vi "Conv AB to enum.vi"(8 "Error In":errorcluster, 11 "Inputs":T2) -> (0 "Error Out":errorcluster, 3 "Input State":T1)   [LabVIEW 2018]
doc: "This VI transforms the input cluster into an enumerated type for specifying the state of the inputs A and B."
uses:
  controls/Cluster for displaying  ABR switch states.ctl
  Enum Defining AB State.ctl
  controls/Enum Defining FSM State.ctl
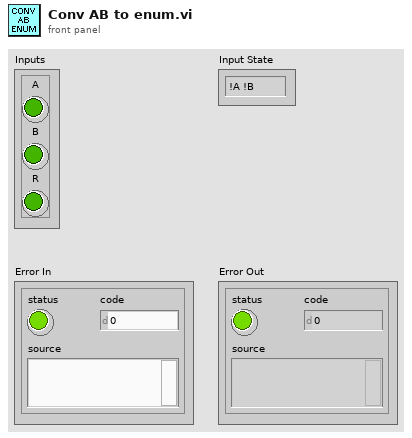
[diagram p1: front panel]
types:
  T1 = typedef "Enum Defining AB State.ctl" = enum16{"!A !B", "!A  B", " A !B", " A B"}
  T2 = typedef "Cluster for displaying  ABR switch states.ctl" = cluster{"A":bool, "B":bool, "R":bool}
  T3 = typedef "Enum Defining FSM State.ctl" = enum16{"S0", "S1", "S2", "S3"}
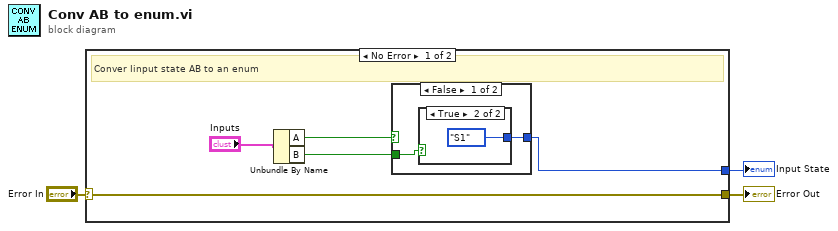
[diagram p0: block diagram]
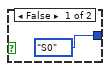
[diagram p2: hidden frame]
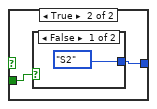
[diagram p3: hidden frame]
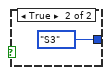
[diagram p4: hidden frame]
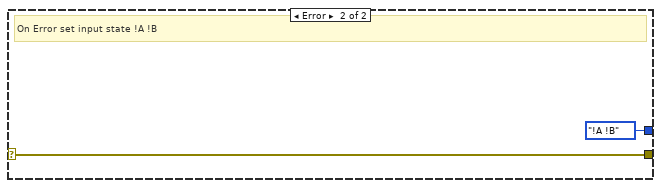
[diagram p5: hidden frame]
diagram:
  n1 = case shown="No Error" "Error In" {
    selector: "Error In" -> [w8 w18]
    tunnel: [w8 w18] -> w2
    tunnel: [w4 Enum_Defining_AB_State."!A !B" ("Input State")] -> w1
    frame No Error {
      # "Conver Iinput state AB to an enum"
      n2 = Unbundle By Name("Inputs") -> ("A"=w6:bool, "B"=w5:bool)
      n3 = case shown="False" w6 {
        tunnel: w5 -> [w10 w14]
        tunnel: [w9 w13] -> w4
        frame False {
          n4 = case shown="True" w10 {
            tunnel: [Enum_Defining_FSM_State."S0" ("Present State") Enum_Defining_FSM_State."S1" ("Present State")] -> w9
            frame False {
            }
            frame True {
            }
          }
        }
        frame True {
          n5 = case shown="False" w14 {
            tunnel: [Enum_Defining_FSM_State."S2" ("Present State") Enum_Defining_FSM_State."S3" ("Present State")] -> w13
            frame False {
            }
            frame True {
            }
          }
        }
      }
    }
    frame Error {
      # "On Error set input state !A !B"
    }
  }
  "Error Out" <- w2
  "Input State" <- w1
